vi "svx_DetermineDecimation.vi"(8 "error in (no error)":errorcluster, 10 "input buffer size":i32, 11 "display width":i32) -> (0 "error out":errorcluster, 1 "no decimation?":bool, 2 "output buffer size":i32, 3 "decimation\nfactor":i32)   [LabVIEW 2017, in "SVX Waterfall Graph.xctl"]
doc: "This VI calculates the decimation factor and display buffer size for a max/min decimation using the <B>sfpCore Specified Max Min Decimate Ixx 1D Array</B> VIs."
uses:
  <vilib>/addons/_XControls/Waterfall Graph/SVX Waterfall Graph.xctl
panel:
  in  "Case Constant\n(See Context Help)":bool=TRUE
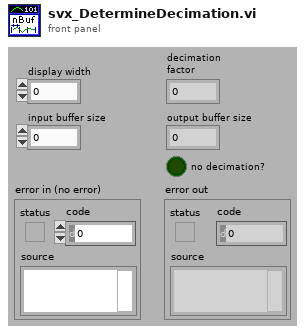
[diagram p1: front panel]
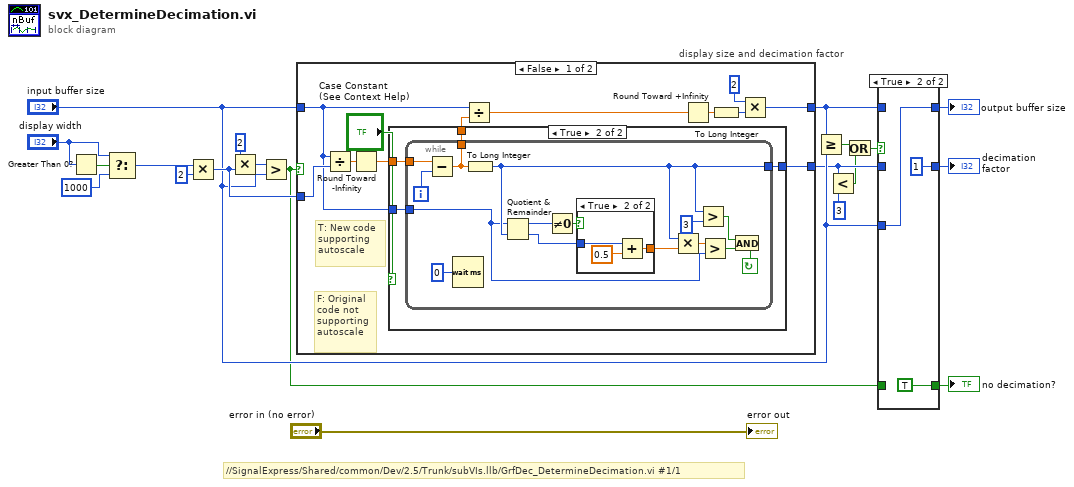
[diagram p0: block diagram]
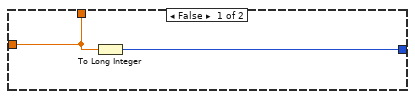
[diagram p3: hidden frame]
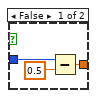
[diagram p4: hidden frame]
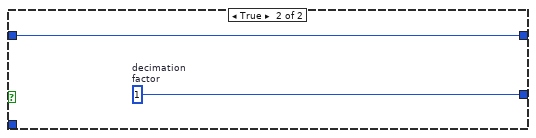
[diagram p5: hidden frame]
diagram:
  # "//SignalExpress/Shared/common/Dev/2.5/Trunk/subVIs.llb/GrfDec_DetermineDecimation.vi #1/1"
  n1 = Greater Than 0?(x="display width") -> (x > 0?=w1:bool)
  n2 = Select(t="display width", s=w1, f=1000) -> (s? t:f=w2:i32)
  n3 = Multiply(x=w2, y=2) -> (x*y=w20:i32)
  n4 = Multiply(x=2, y=w20) -> (x*y=w19:i32)
  n5 = Greater?(x=w19, y="input buffer size") -> (0:w5:bool)
  n6 = case "display size and decimation factor" shown="False" w5 {
    tunnel: "input buffer size" -> [w25 w61]
    tunnel: w20 -> [w32 _]
    tunnel: [w27 w61] -> w14
    tunnel: [w24 w60] -> w10
    frame False {
      # "F: Original\ncode not\nsupporting\nautoscale"
      # "T: New code\nsupporting\nautoscale"
      n7 = Divide(x=w25, y=w32) -> (x/y=w31:dbl)
      n8 = Round Toward -Infinity(1:w31) -> (0:w23:dbl)
      n9 = case shown="True" "Case Constant\n(See Context Help)" {
        tunnel: w25 -> [_ w38]
        tunnel: [w33 w37] -> w24
        tunnel: w23 -> [w34 w36]
        tunnel: [w34 w35] -> w22
        frame False {
          n10 = To Long Integer(number=w34) -> (32bit integer=w33:i32)
        }
        frame True {
          n11 = while {
            tunnel: w36 -> [w45]
            tunnel: w38 -> [w39]
            tunnel: [w50] -> w37
            tunnel: [w43] -> w35
            i -> [w44]
            stop <- w46 continue-if-true
            n12 = Subtract(x=w45, y=w44) -> (x-y=w43:dbl)
            n13 = Wait (ms)(milliseconds to wait=u32 0) -> ()  [unwired: 1 out]
            n14 = To Long Integer(number=w43) -> (32bit integer=w50:i32)
            n15 = Quotient & Remainder(x=w39, y=w50) -> (x-y*floor(x/y)=w52:i32, floor(x/y)=w40:i32)
            n16 = Not Equal To 0?(x=w52) -> (x != 0?=w53:bool)
            n17 = case shown="True" w53 {
              tunnel: [w54 w57] -> w41
              tunnel: w40 -> [w55 w58]
              frame False {
                n18 = Subtract(x=w55, y=0.5) -> (x-y=w54:dbl)
              }
              frame True {
                n19 = Add(x=w58, y=0.5) -> (x+y=w57:dbl)
              }
            }
            n20 = Multiply(x=w50, y=w41) -> (x*y=w51:dbl)
            n21 = Greater?(x=w50, y=3) -> (0:w48:bool)
            n22 = Greater?(x=w51, y=w39) -> (0:w47:bool)
            n23 = And(x=w48, y=w47) -> (x .and. y?=w46:bool)
          }
        }
      }
      n24 = Divide(x=w25, y=w22) -> (x/y=w30:dbl)
      n25 = Round Toward +Infinity(x=w30) -> (ceil(x): smallest int >= x=w29:dbl)
      n26 = To Long Integer(number=w29) -> (32bit integer=w28:i32)
      n27 = Multiply(x=2, y=w28) -> (x*y=w27:i32)
    }
    frame True {
      w60 = 1  # decimation factor
    }
  }
  n28 = Greater Or Equal?(x=w14, y="input buffer size") -> (x >= y?=w7:bool)
  n29 = Less?(x=w10, y=3) -> (x < y?=w6:bool)
  n30 = Or(x=w7, y=w6) -> (x .or. y?=w8:bool)
  n31 = case shown="True" w8 {
    tunnel: "input buffer size" -> [_ w65]
    tunnel: w14 -> [w64 _]
    tunnel: [w64 w65] -> w13
    tunnel: w10 -> [w63 _]
    tunnel: [w63 1 ("decimation\nfactor")] -> w12
    tunnel: w5 -> [w62 _]
    tunnel: [w62 TRUE] -> w11
    frame False {
    }
    frame True {
    }
  }
  "decimation\nfactor" <- w12
  "output buffer size" <- w13
  "no decimation?" <- w11
  "error out" <- "error in (no error)"
